vi "test Parse Sorted Object Dictionary_1.vi"(11 "Test Case In":refnum<class "test EDS.lvclass">) -> (0 "error out":errorcluster, 3 "Test Case Out":refnum<class "test EDS.lvclass">)   [LabVIEW 2024, in "test EDS.lvclass"]
uses:
  test EDS.lvclass
  Core/EDS/EDS.lvclass
  Core/Object Type.ctl
  Core/Data Type.ctl
  Core/Access Type.ctl
  Core/EDS/EDS.lvclass/EDS.ctl
  <vilib>/Astemes/LUnit/Test Case.lvclass/Test Case.ctl
  <vilib>/Astemes/LUnit/Append Fail Result.vi
  <vilib>/Astemes/LUnit/Append Pass Result.vi
  <vilib>/Astemes/LUnit/Run In UI.vi
  <vilib>/Utility/error.llb/Clear Errors.vi
  Core/OD Sub-Entry/OD Sub-Entry.lvclass
  <vilib>/Astemes/LUnit/Test Case.lvclass
  Core/EDS.lvlib
  Core/OD Entry/OD Entry.lvclass
  Core/Sorted Object Dictionary/Sorted Object Dictionary.lvclass
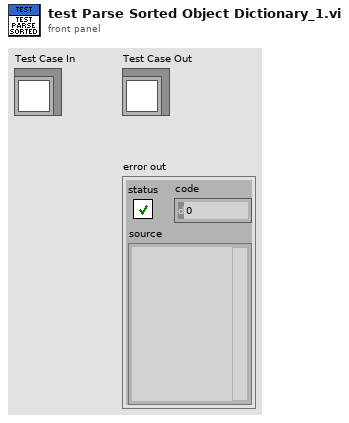
[diagram p1: front panel]
types:
  T1 = typedef "EDS.lvlib/Access Type.ctl" = enum16{"ro", "wo", "rw", "rwr", "rww", "const"}
  T2 = typedef "EDS.lvlib/Data Type.ctl" = u16
  T3 = typedef "EDS.lvlib/Object Type.ctl" = u8
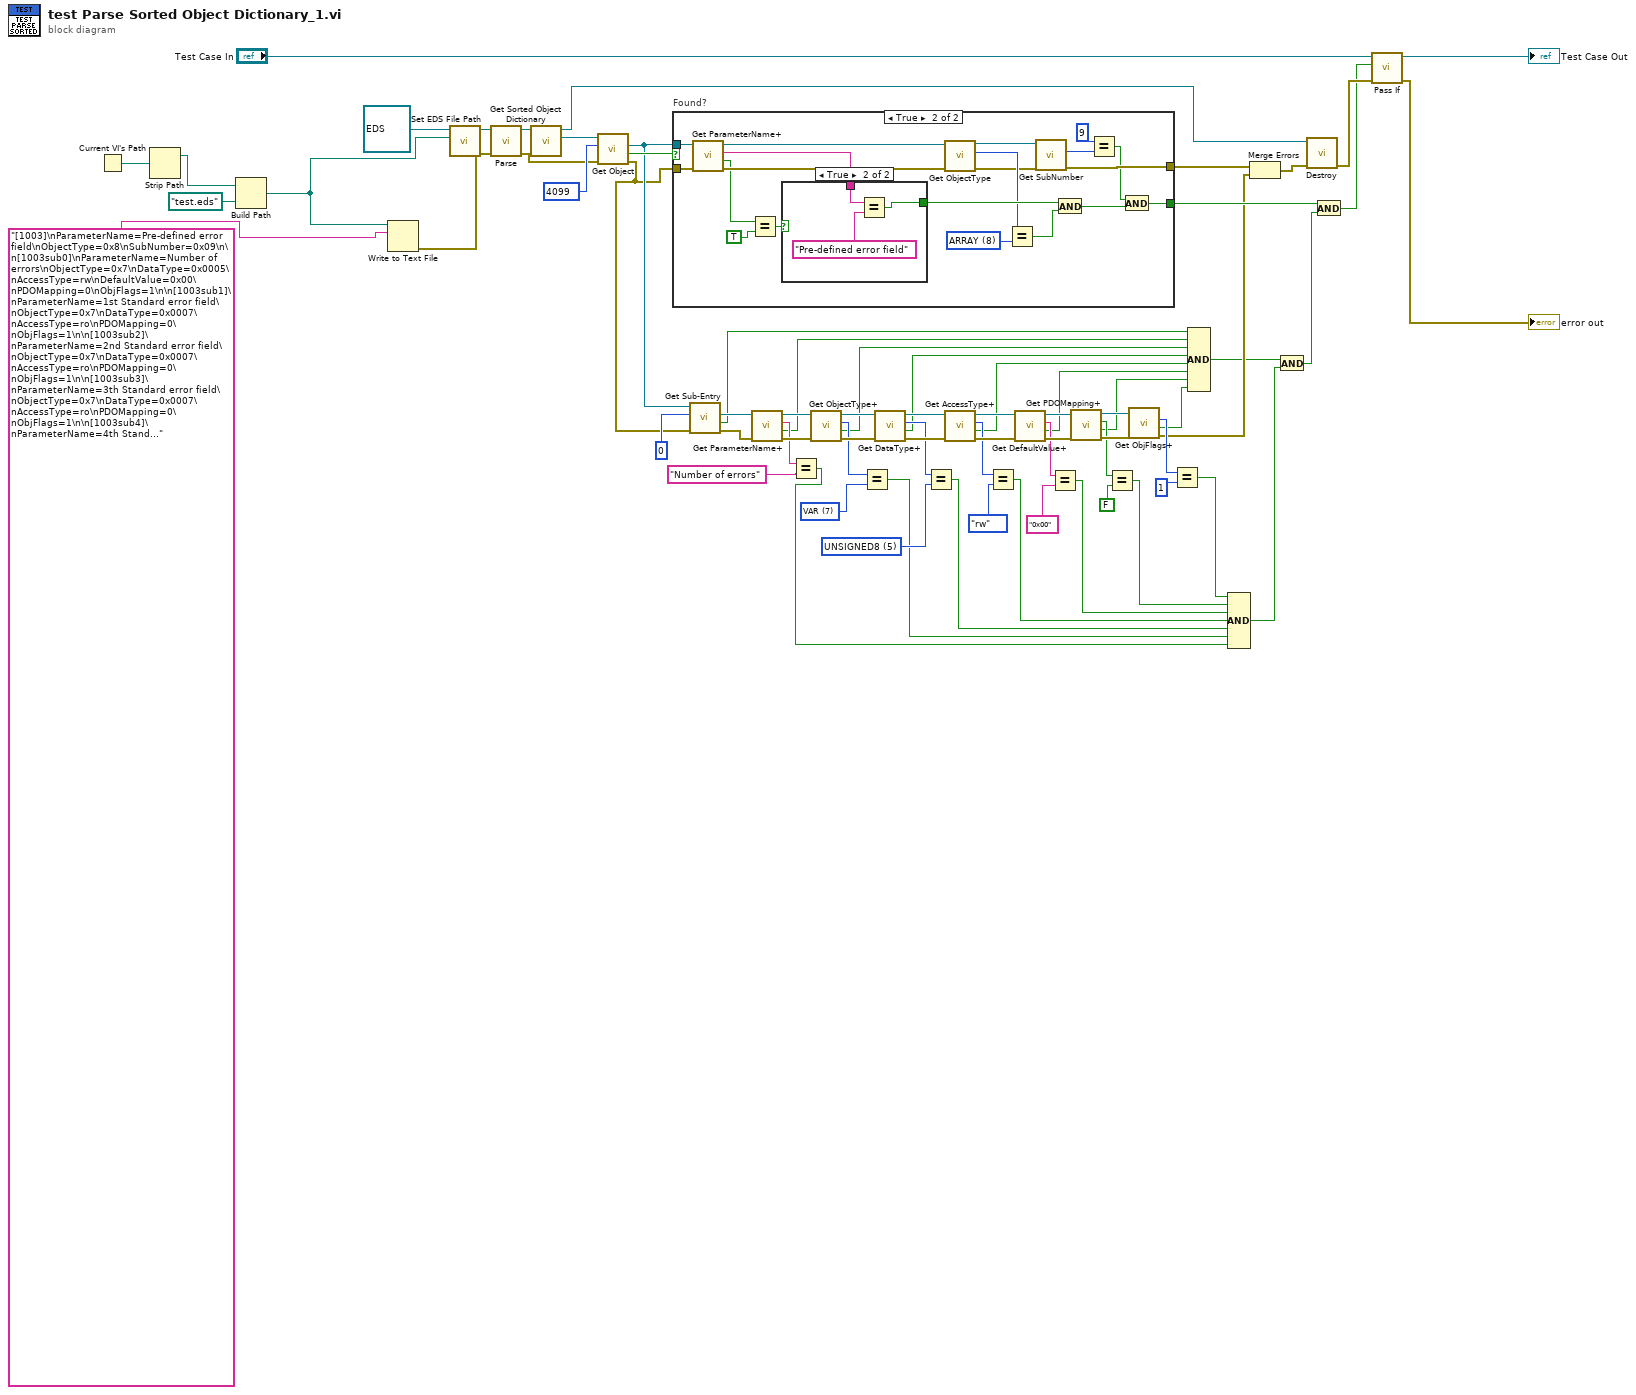
[diagram p0: block diagram]
diagram:
  w36 = T2 5 items=["BOOLEAN"=1, "INTEGER8"=2, "INTEGER16"=3, "INTEGER32"=4, "UNSIGNED8"=5, "UNSIGNED16"=6, "UNSIGNED32"=7, "REAL32"=8, "VISIBLE_STRING"=9, "OCTET_STRING"=10, "UNICODE_STRING"=11, "TIME_OF_DAY"=12, "TIME_DIFFERENCE"=13, "RESERVED1"=14, "DOMAIN"=15, "INTEGER24"=16, "REAL64"=17, "INTEGER40"=18, "INTEGER48"=19, "INTEGER56"=20, "INTEGER64"=21, "UNSIGNED24"=22, "RESERVED2"=23, "UNSIGNED40"=24, "UNSIGNED48"=25, "UNSIGNED56"=26, "UNSIGNED64"=27, "RESERVED3"=28, "RESERVED4"=29, "RESERVED5"=30, "RESERVED6"=31, "PDO_COMMUNICATION_PARAMETER"=32, "PDO_MAPPING"=33, "SDO_PARAMETER"=34, "IDENTITY"=35, "RESERVED7"=36] ("DataType")
  w38 = T3 7 items=["NULL"=0, "DOMAIN"=2, "DEFTYPE"=5, "DEFSTRUCT"=6, "VAR"=7, "ARRAY"=8, "RECORD"=9] ("ObjectType")
  n1 = Current VI's Path() -> (path=w67:path)
  n2 = Strip Path(path=w67) -> (stripped path=w63:path)  [unwired: 1 out]
  n3 = Build Path(base path=w63, name or relative path=path "test.eds") -> (appended path=w64:path)
  n4 = Write to Text File(file (use dialog)=w64, text="[1003]\nParameterName=Pre-defined error field\nObjectType=0x8\nSubNumber=0x09\n\n[1003sub0]\nParameterName=Number of errors\nObjectType=0x7\nDataType=0x0005\nAccessType=rw\nDefaultValue=0x00\nPDOMapping=0\nObjFlags=1\n\n[1003sub1]\nParameterName=1st Standard error field\nObjectType=0x7\nDataType=0x0007\nAccessType=ro\nPDOMapping=0\nObjFlags=1\n\n[1003sub2]\nParameterName=2nd Standard error field\nObjectType=0x7\nDataType=0x0007\nAccessType=ro\nPDOMapping=0\nObjFlags=1\n\n[1003sub3]\nParameterName=3th Standard error field\nObjectType=0x7\nDataType=0x0007\nAccessType=ro\nPDOMapping=0\nObjFlags=1\n\n[1003sub4]\nParameterName=4th Standard error field\nObjectType=0x7\nDataType=0x0007\nAccessType=ro\nPDOMapping=0\nObjFlags=1\n\n[1003sub5]\nParameterName=5th Standard error field\nObjectType=0x7\nDataType=0x0007\nAccessType=ro\nPDOMapping=0\nObjFlags=1\n\n[1003sub6]\nParameterName=6th Standard error field\nObjectType=0x7\nDataType=0x0007\nAccessType=ro\nPDOMapping=0\nObjFlags=1\n\n[1003sub7]\nParameterName=7th Standard error field\nObjectType=0x7\nDataType=0x0007\nAccessType=ro\nPDOMapping=0\nObjFlags=1\n\n[1003sub8]\nParameterName=8th Standard error field\nObjectType=0x7\nDataType=0x0007\nAccessType=ro\nPDOMapping=0\nObjFlags=1") -> (error out=w65:errorcluster)  [unwired: 2 in, 2 out]
  n5 = call "Set EDS File Path.vi"("EDS File Path"=w64, "EDS in"=refnum<class "EDS.lvclass"> refnum ("EDS.lvlib:EDS.lvclass")) -> ("EDS out"=w68:refnum<class "EDS.lvclass">)  [unwired: 9 in]
  n6 = call "Parse.vi"("error in"=w65, "EDS in"=w68) -> ("error out"=w9:errorcluster, "EDS out"=w62:refnum<class "EDS.lvclass">)  [unwired: 8 in]
  n7 = call "Get Sorted Object Dictionary.vi"("EDS in"=w62) -> ("Sorted Object Dictionary"=w59:refnum<class "Sorted Object Dictionary.lvclass">, "EDS out"=w61:refnum<class "EDS.lvclass">)  [unwired: 9 in]
  n8 = call "Get Object.vi"("error in"=w9, "Index"=u16 4099 ("Numeric"), "Sorted Object Dictionary in"=w59) -> ("error out"=w8:errorcluster, "Found?"=w55:bool, "OD Entry"=w54:refnum<class "OD Entry.lvclass">)  [unwired: 5 in, 1 out]
  n9 = case "Found?" shown="True" w55 {
    selector: w55 -> [w73 _]
    tunnel: w54 -> [_ w94]
    tunnel: w8 -> [w74 w93]
    tunnel: [w73 w77] -> w58
    tunnel: [w74 w81] -> w56
    frame False {
    }
    frame True {
      w85 = T3 8 items=["NULL"=0, "DOMAIN"=2, "DEFTYPE"=5, "DEFSTRUCT"=6, "VAR"=7, "ARRAY"=8, "RECORD"=9] ("y")
      n10 = call "Get ParameterName+.vi"("Error In"=w93, "reference in"=w94) -> ("Error Out"=w87:errorcluster, "Defined?"=w75:bool, "ParameterName"=w91:string, "reference out"=w88:refnum<class "OD Entry.lvclass">)  [unwired: 6 in]
      n11 = Equal?(x=w75, y=TRUE) -> (x = y?=w90:bool)
      n12 = case shown="True" w90 {
        selector: w90 -> [w95 _]
        tunnel: w91 -> [_ w98]
        tunnel: [w95 w96] -> w89
        frame False {
        }
        frame True {
          n13 = Equal?(x=w98, y="Pre-defined error field") -> (x = y?=w96:bool)
        }
      }
      n14 = call "Get ObjectType.vi"("Error In"=w87, "reference in"=w88) -> ("Error Out"=w82:errorcluster, "ObjectType"=w86:T3, "reference out"=w80:refnum<class "OD Entry.lvclass">)  [unwired: 7 in]
      n15 = Equal?(x=w86, y=w85) -> (x = y?=w83:bool)
      n16 = call "Get SubNumber.vi"("Error In"=w82, "reference in"=w80) -> ("Error Out"=w81:errorcluster, "SubNumber"=w79:u8)  [unwired: 6 in, 2 out]
      n17 = And(x=w89, y=w83) -> (x .and. y?=w84:bool)
      n18 = Equal?(x=u8 9, y=w79) -> (x = y?=w76:bool)
      n19 = And(x=w76, y=w84) -> (x .and. y?=w77:bool)
    }
  }
  n20 = call "Get Sub-Entry.vi"("Error In"=w8, "Sub-Index"=u8 0, "reference in"=w54) -> ("Error Out"=w52:errorcluster, "Found?"=w40:bool, "OD Sub-Entry"=w53:refnum<class "OD Sub-Entry.lvclass">)  [unwired: 5 in, 1 out]
  n21 = call "Get ParameterName+.vi"("Error In"=w52, "reference in"=w53) -> ("Error Out"=w51:errorcluster, "Defined?"=w7:bool, "ParameterName"=w42:string, "reference out"=w50:refnum<class "OD Sub-Entry.lvclass">)  [unwired: 6 in]
  n22 = Equal?(x=w42, y="Number of errors") -> (x = y?=w17:bool)
  n23 = call "Get ObjectType+.vi"("Error In"=w51, "reference in"=w50) -> ("Error Out"=w48:errorcluster, "Defined?"=w6:bool, "ObjectType"=w39:T3, "reference out"=w49:refnum<class "OD Sub-Entry.lvclass">)  [unwired: 6 in]
  n24 = Equal?(x=w39, y=w38) -> (x = y?=w16:bool)
  n25 = call "Get DataType+.vi"("Error In"=w48, "reference in"=w49) -> ("Error Out"=w45:errorcluster, "Defined?"=w5:bool, "DataType"=w37:T2, "reference out"=w46:refnum<class "OD Sub-Entry.lvclass">)  [unwired: 6 in]
  n26 = Equal?(x=w37, y=w36) -> (x = y?=w15:bool)
  n27 = call "Get AccessType+.vi"("Error In"=w45, "reference in"=w46) -> ("Error Out"=w43:errorcluster, "Defined?"=w4:bool, "AccessType"=w35:T1, "reference out"=w44:refnum<class "OD Sub-Entry.lvclass">)  [unwired: 6 in]
  n28 = Equal?(x=w35, y=Access_Type."rw") -> (x = y?=w14:bool)
  n29 = call "Get DefaultValue+.vi"("Error In"=w43, "reference in"=w44) -> ("Error Out"=w32:errorcluster, "Defined?"=w3:bool, "DefaultValue"=w29:string, "reference out"=w33:refnum<class "OD Sub-Entry.lvclass">)  [unwired: 6 in]
  n30 = Equal?(x=w29, y="0x00") -> (x = y?=w13:bool)
  n31 = call "Get PDOMapping+.vi"("Error In"=w32, "reference in"=w33) -> ("Error Out"=w30:errorcluster, "Defined?"=w2:bool, "PDOMapping"=w27:bool, "reference out"=w31:refnum<class "OD Sub-Entry.lvclass">)  [unwired: 6 in]
  n32 = Equal?(x=w27, y=FALSE) -> (x = y?=w12:bool)
  n33 = call "Get ObjFlags+.vi"("Error In"=w30, "reference in"=w31) -> ("Error Out"=w23:errorcluster, "Defined?"=w1:bool, "ObjFlags"=w25:u32)  [unwired: 6 in, 1 out]
  n34 = Equal?(x=w25, y=u32 1) -> (x = y?=w11:bool)
  n35 = Compound Arithmetic op=AND(w40, w7, w6, w5, w4, w3, w2, w1) -> (w21:bool)
  n36 = Compound Arithmetic op=AND(w11, w12, w13, w14, w15, w16, w17) -> (w18:bool)
  n37 = Merge Errors(w56, w23) -> (w24:errorcluster)
  n38 = And(x=w21, y=w18) -> (x .and. y?=w19:bool)
  n39 = call "Destroy.vi"("error in"=w24, "EDS in"=w61) -> ("error out"=w57:errorcluster)  [unwired: 8 in, 1 out]
  n40 = And(x=w58, y=w19) -> (x .and. y?=w22:bool)
  n41 = call <vilib>:"Pass If.vi"("error in (no error)"=w57, "Pass?"=w22, "LUnit Test Case In"="Test Case In") -> ("error out"=→"error out":errorcluster, "LUnit Test Case Out"=→"Test Case Out":refnum<class "test EDS.lvclass">)  [unwired: 7 in]
